vi "Derivative LFR cycles (SubVI).vi"(8 "Derivative LPF cutoff (Hz)":dbl=15.0, 9 "Derivative filter on?":bool=TRUE, 10 "dt":dbl=50.0, 11 "Waveform (samples) in":dbl[](array[numeric])) -> (0 "Fourth derivative (samples)":dbl[](array[numeric]), 1 "Second derivative (samples)":dbl[](array[numeric]), 2 "First derivative (samples)":dbl[](array[numeric]), 3 "Waveform (samples) out":dbl[](array[numeric]))   [LabVIEW 2017]
uses:
  <vilib>/Analysis/NI_AALPro.lvlib
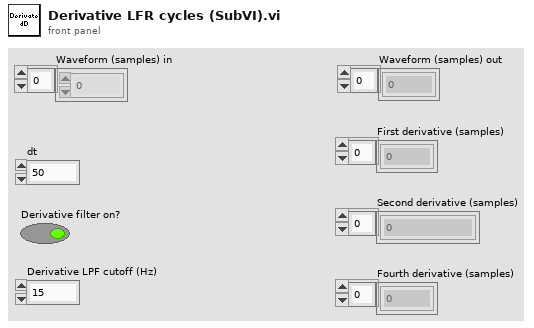
[diagram p1: front panel]
types:
  T1 = enum32{"Lowpass", "Highpass", "Bandpass", "Bandstop"}
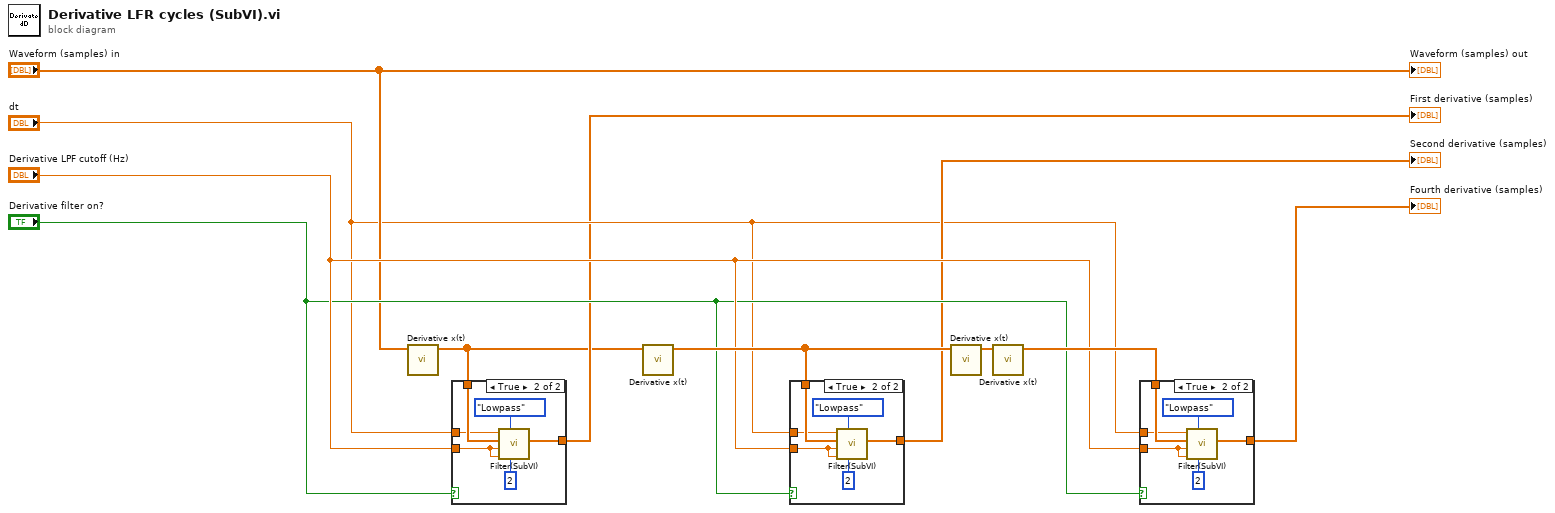
[diagram p0: block diagram]
diagram:
  n1 = call <vilib>:"Derivative x(t).vi"("X"="Waveform (samples) in") -> ("dX/dt"=w1:dbl[])  [unwired: 9 in, 1 out]
  n2 = case shown="True" "Derivative filter on?" {
    tunnel: w1 -> [w12 w16]
    tunnel: "dt" -> [_ w15]
    tunnel: "Derivative LPF cutoff (Hz)" -> [_ w14]
    tunnel: [w12 w13] -> w2
    frame False {
    }
    frame True {
      n3 = call "Filter(SubVI).vi"("order"=2, "filter type"=T1."Lowpass", "low cutoff freq: fl"=w14, "high cutoff freq: fh"=w14, "Data"=w16, "dt"=w15) -> ("Filtered Data"=w13:dbl[])  [unwired: 5 in]
    }
  }
  "First derivative (samples)" <- w2
  n4 = call <vilib>:"Derivative x(t).vi"("X"=w1) -> ("dX/dt"=w9:dbl[])  [unwired: 9 in, 1 out]
  n5 = case shown="True" "Derivative filter on?" {
    tunnel: w9 -> [w19 w23]
    tunnel: "dt" -> [_ w22]
    tunnel: "Derivative LPF cutoff (Hz)" -> [_ w21]
    tunnel: [w19 w20] -> w5
    frame False {
    }
    frame True {
      n6 = call "Filter(SubVI).vi"("order"=2, "filter type"=T1."Lowpass", "low cutoff freq: fl"=w21, "high cutoff freq: fh"=w21, "Data"=w23, "dt"=w22) -> ("Filtered Data"=w20:dbl[])  [unwired: 5 in]
    }
  }
  "Second derivative (samples)" <- w5
  n7 = call <vilib>:"Derivative x(t).vi"("X"=w9) -> ("dX/dt"=w11:dbl[])  [unwired: 9 in, 1 out]
  n8 = call <vilib>:"Derivative x(t).vi"("X"=w11) -> ("dX/dt"=w10:dbl[])  [unwired: 9 in, 1 out]
  n9 = case shown="True" "Derivative filter on?" {
    tunnel: w10 -> [w26 w30]
    tunnel: "dt" -> [_ w29]
    tunnel: "Derivative LPF cutoff (Hz)" -> [_ w28]
    tunnel: [w26 w27] -> w4
    frame False {
    }
    frame True {
      n10 = call "Filter(SubVI).vi"("order"=2, "filter type"=T1."Lowpass", "low cutoff freq: fl"=w28, "high cutoff freq: fh"=w28, "Data"=w30, "dt"=w29) -> ("Filtered Data"=w27:dbl[])  [unwired: 5 in]
    }
  }
  "Fourth derivative (samples)" <- w4
  "Waveform (samples) out" <- "Waveform (samples) in"
